vi "Do.vi"(8 "error in (no error)":errorcluster, 9 "Events":refnum<class "Events.lvclass">, 10 "Message Loop Data in":T4, 11 "Error JSON2 in":refnum<class "Error JSON.lvclass">) -> (0 "error out":errorcluster, 1 "Write request":T12, 2 "Message Loop Data out":T4, 3 "Error JSON2 out":refnum<class "Error JSON.lvclass">)   [LabVIEW 2020, in "wamplv.lvlib" / "Error JSON.lvclass"]
uses:
  Error JSON.lvclass
  Utils/Utils.lvclass
  TypeDefs/WAMP Message Codes.ctl
  wamplv.lvlib
  4bcbb7f0-c468-459d-b905-e591281fd257.vi
  WAMP Client/Private/TypeDef/Publish Requests Map.ctl
  WAMP Client/Private/TypeDef/Endpoint Data.ctl
  Call/ICallRequest/ICallRequest.lvclass
  WAMP Client/Private/TypeDef/CALL Request Map.ctl
  WAMP Client/Private/TypeDef/SUBSCRIBE Requests Map.ctl
  WAMP Client/Private/TypeDef/Subscriptions Map.ctl
  WAMP Client/Private/TypeDef/Unsubscribe Requests Map.ctl
  WAMP Client/Private/TypeDef/Unregister requests map.ctl
  WAMP Client/Private/TypeDef/Message Loop Data.ctl
  TypeDefs/Transport type.ctl
  WAMP Client/Private/TypeDef/Write queue item.ctl
  Events/EventsParent/Events.lvclass
  Subscribe/ISubscribe/ISubscribe.lvclass
  Publish/IPublish/IPublish.lvclass
  Message loop classes/Subscription details/SubscriptionDetailsParent/SubscriptionDetailsParent.lvclass
  Unsubscribe/IUnsubscribe/IUnsubscribe.lvclass
  Register/IRegister/IRegister.lvclass
  Unregister/IUnregister/IUnregister.lvclass
  WAMP Client/API/TypeDefs/Error or abort detail (JSON).ctl
  WAMP Client/Private/TypeDef/Error (JSON).ctl
panel:
  in  "Error Request":T1
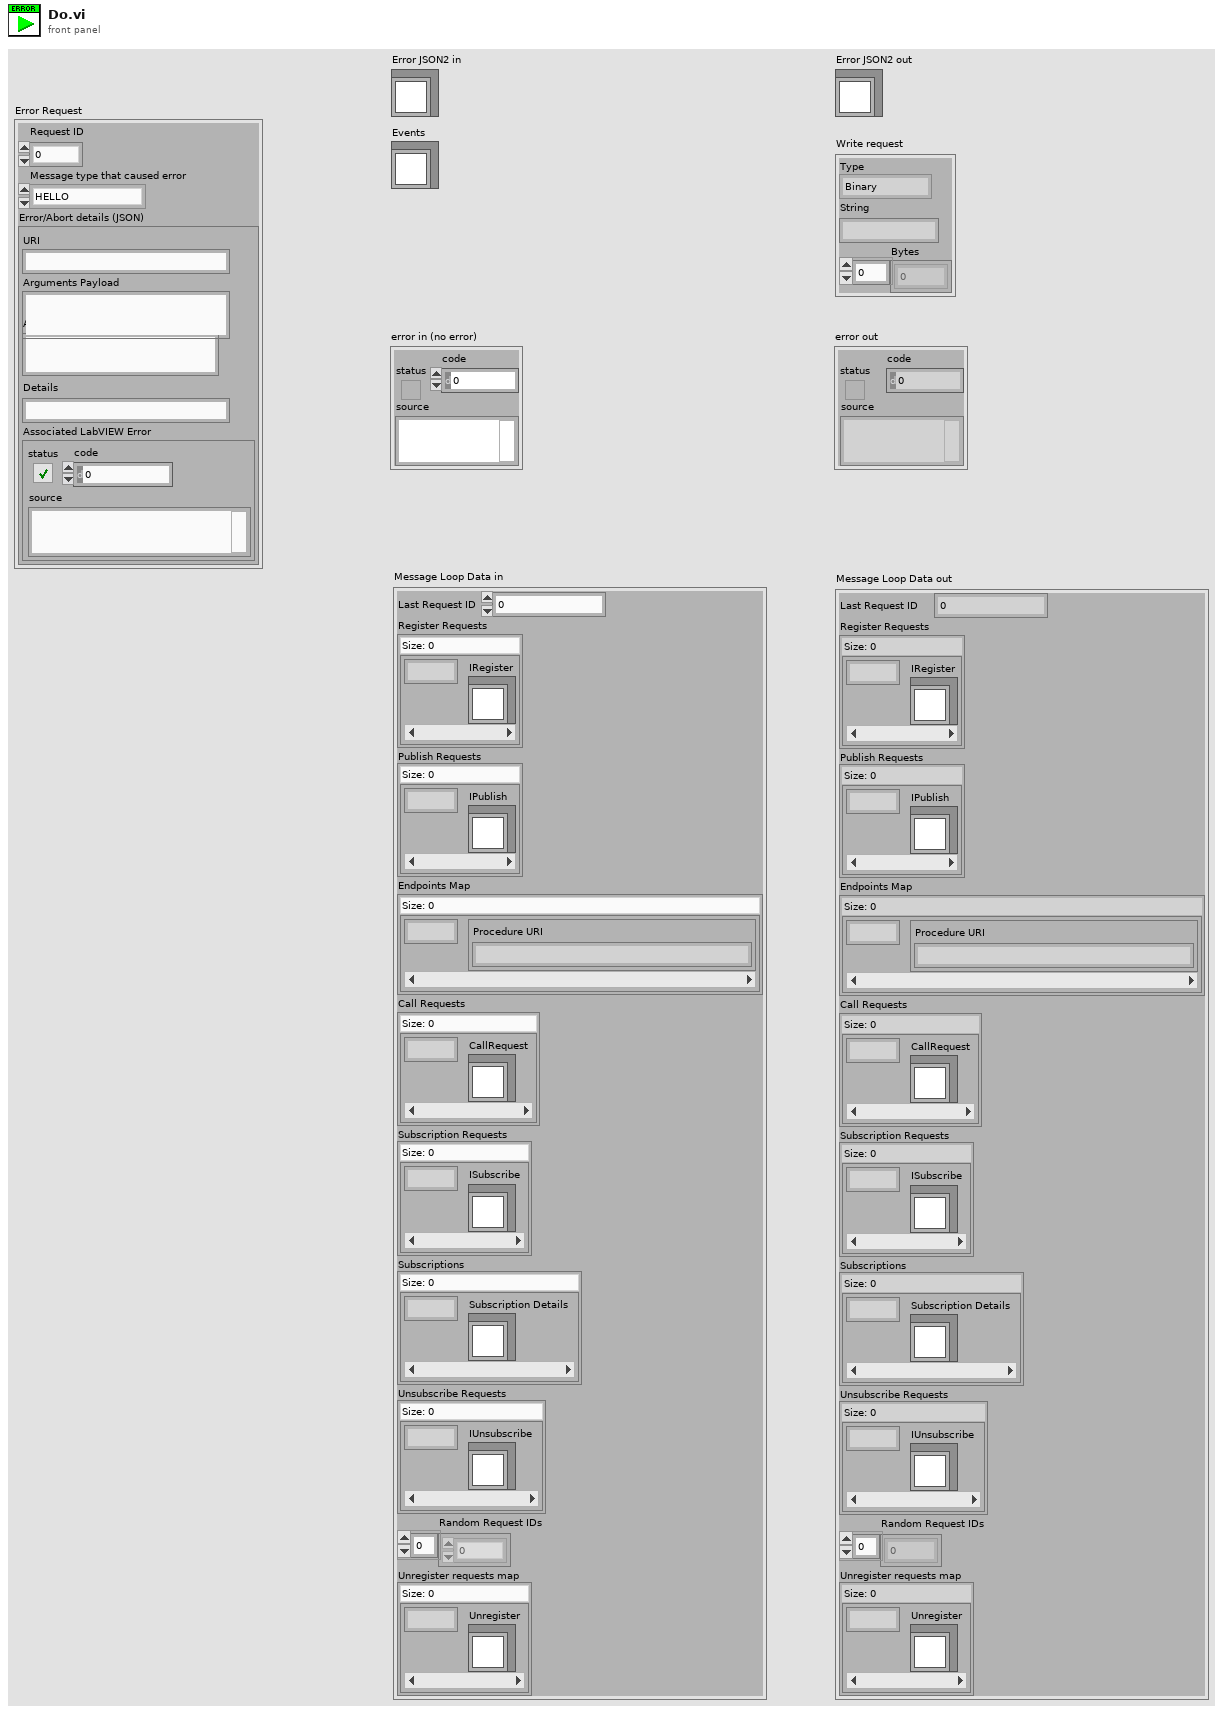
[diagram p1: front panel]
types:
  T1 = typedef "wamplv.lvlib/Error (JSON).ctl" = cluster{"Request ID":u64, "Message type that caused error":T2, "Error/Abort details (JSON)":T3}
  T2 = typedef "wamplv.lvlib/WAMP Message Codes.ctl" = enum8{"HELLO", "WELCOME", "CHALLENGE", "AUTHENTICATE", "ABORT", "GOODBYE", "ERROR", "PUBLISH", "PUBLISHED", "SUBSCRIBE", "SUBSCRIBED", "UNSUBSCRIBE", "UNSUBSCRIBED", "EVENT", "CALL", "RESULT", "REGISTER", "REGISTERED", "UNREGISTER", "UNREGISTERED", "INVOCATION", "YIELD"}
  T3 = typedef "wamplv.lvlib/Error or abort detail (JSON).ctl" = cluster{"URI":string, "Arguments Payload":string, "ArgumentKw Payload":string, "Details":string, "Associated LabVIEW Error":errorcluster}
  T4 = typedef "wamplv.lvlib/Message Loop Data.ctl" = cluster{"Last Request ID":u64, "Register Requests":map{u64, refnum<class "IRegister.lvclass">}, "Publish Requests":T5, "Endpoints Map":map{u64, T6}, "Call Requests":T7, "Subscription Requests":T8, "Subscriptions":T9, "Unsubscribe Requests":T10, "Random Request IDs":u64[], "Unregister requests map":T11}
  T5 = typedef "wamplv.lvlib/Publish Requests Map.ctl" = map{u64, refnum<class "IPublish.lvclass">}
  T6 = typedef "wamplv.lvlib/Endpoint Data.ctl" = cluster{"Procedure URI":string}
  T7 = typedef "wamplv.lvlib/CALL Request Map.ctl" = map{u64, refnum<class "ICallRequest.lvclass">}
  T8 = typedef "wamplv.lvlib/SUBSCRIBE Requests Map.ctl" = map{u64, refnum<class "ISubscribe.lvclass">}
  T9 = typedef "wamplv.lvlib/Subscriptions Map.ctl" = map{u64, refnum<class "SubscriptionDetailsParent.lvclass">}
  T10 = typedef "wamplv.lvlib/Unsubscribe Requests Map.ctl" = map{u64, refnum<class "IUnsubscribe.lvclass">}
  T11 = typedef "wamplv.lvlib/Unregister requests map.ctl" = map{u64, refnum<class "IUnregister.lvclass">}
  T12 = typedef "wamplv.lvlib/Write queue item.ctl" = cluster{"Type":T13, "String":string, "Bytes":u8[]}
  T13 = typedef "wamplv.lvlib/Transport type.ctl" = enum16{"Binary", "Text"}
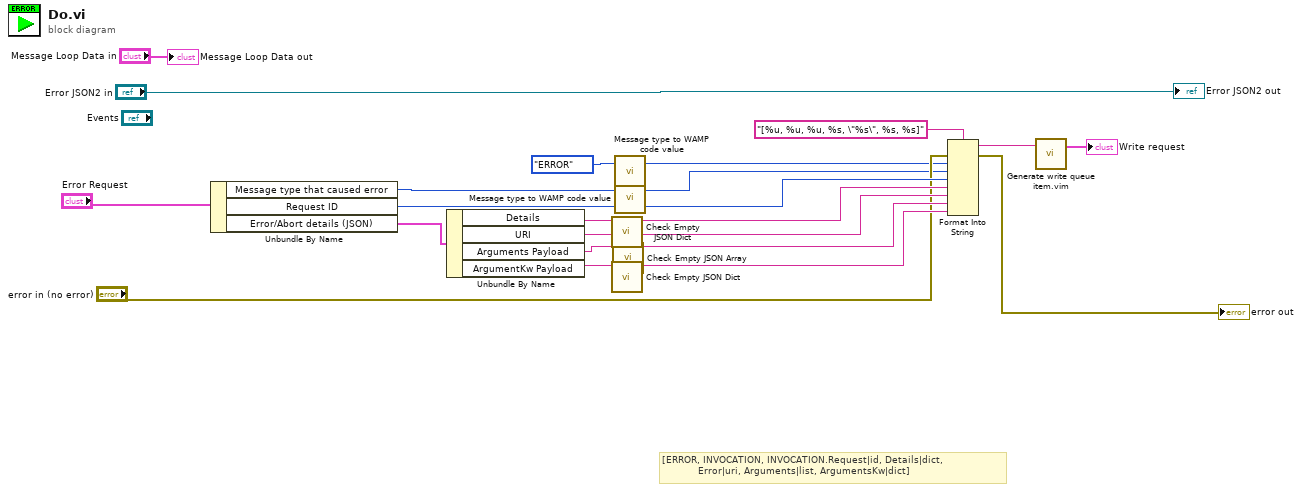
[diagram p0: block diagram]
diagram:
  # "[ERROR, INVOCATION, INVOCATION.Request|id, Details|dict,\n            Error|uri, Arguments|list, ArgumentsKw|dict]"
  n1 = Unbundle By Name("Error Request") -> ("Message type that caused error"=w2:T2, "Request ID"=w11:u64, "Error/Abort details (JSON)"=w12:T3)
  n2 = Unbundle By Name(w12) -> ("Details"=w14:string, "URI"=w13:string, "Arguments Payload"=w19:string, "ArgumentKw Payload"=w16:string)
  n3 = call "Check Empty JSON Dict.vi"("JSON in"=w14) -> ("JSON out"=w15:string)  [unwired: 10 in]
  n4 = call "Check Empty JSON Dict.vi"("JSON in"=w16) -> ("JSON out"=w17:string)  [unwired: 10 in]
  n5 = call "Check Empty JSON Array.vi"("JSON in"=w19) -> ("JSON out"=w20:string)  [unwired: 10 in]
  n6 = call "Message type to WAMP code value.vi"("Message Type"=WAMP_Message_Codes."ERROR" ("Message Codes")) -> ("WAMP Numeric value"=w3:u8)  [unwired: 2 in]
  n7 = call "Message type to WAMP code value.vi"("Message Type"=w2) -> ("WAMP Numeric value"=w1:u8)  [unwired: 2 in]
  n8 = Format Into String(format string="[%u, %u, %u, %s, \"%s\", %s, %s]" ("element"), error in="error in (no error)", w3, w1, w11, w15, w13, w20, w17) -> (resulting string=w6:string, error out=→"error out":errorcluster)  [unwired: 1 in]
  n9 = call "Generate write queue item.vim"("Input"=w6) -> ("Ouput"=→"Write request":T12)  [unwired: 2 in]
  "Error JSON2 out" <- "Error JSON2 in"
  "Message Loop Data out" <- "Message Loop Data in"
